vi "CharToByte(SubVI).vi"(9 "use char":bool, 10 "input u8":u8, 11 "input char":string) -> (1 "output asc":u8, 2 "output char":string, 3 "output u8":u8)   [LabVIEW 2012]
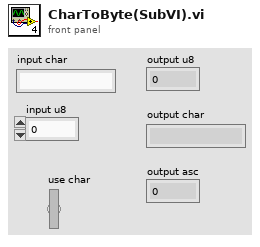
[diagram p1: front panel]
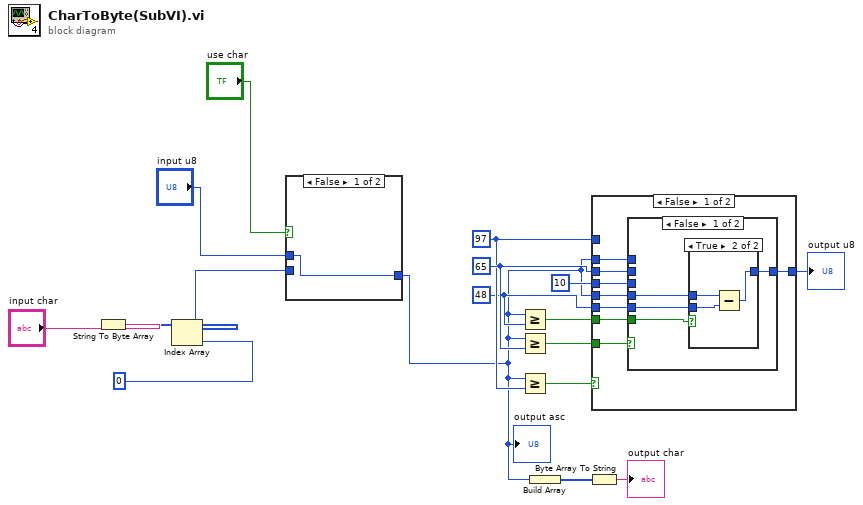
[diagram p0: block diagram]
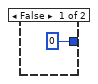
[diagram p3: hidden frame]
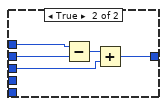
[diagram p4: hidden frame]
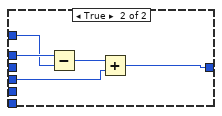
[diagram p5: hidden frame]
diagram:
  w13 = 48
  w17 = 65
  w16 = 97
  n1 = String To Byte Array(string="input char") -> (unsigned byte array=w7:u8[])
  n2 = Index Array(array=w7, index=0) -> (element=w3:u8)
  n3 = case shown="False" "use char" {
    tunnel: w3 -> [_ w19]
    tunnel: [w18 w19] -> w2
    tunnel: "input u8" -> [w18 _]
    frame False {
    }
    frame True {
    }
  }
  "output asc" <- w2
  n4 = Greater Or Equal?(x=w2, y=w13) -> (x >= y?=w12:bool)
  n5 = Greater Or Equal?(x=w2, y=w17) -> (x >= y?=w14:bool)
  n6 = Greater Or Equal?(x=w2, y=w16) -> (x >= y?=w15:bool)
  n7 = Build Array(w2) -> (w11:u8[])
  n8 = Byte Array To String(unsigned byte array=w11) -> (string=→"output char":string)
  n9 = case shown="False" w15 {
    tunnel: w14 -> [w27 _]
    tunnel: w12 -> [w26 _]
    tunnel: w2 -> [w20 w45]
    tunnel: w16 -> [_ w44]
    tunnel: 10 -> [w22 w43]
    tunnel: [w25 w41] -> w6
    tunnel: w2 -> [w24 _]
    tunnel: w13 -> [w23 _]
    tunnel: w17 -> [w21 _]
    frame False {
      n10 = case shown="False" w27 {
        tunnel: w26 -> [w31 _]
        tunnel: [w30 w40] -> w25
        tunnel: w24 -> [w29 _]
        tunnel: w23 -> [w28 _]
        tunnel: w22 -> [_ w39]
        tunnel: w21 -> [_ w37]
        tunnel: w20 -> [_ w36]
        frame False {
          n11 = case shown="True" w31 {
            tunnel: [0 w33] -> w30
            tunnel: w29 -> [_ w35]
            tunnel: w28 -> [_ w34]
            frame False {
            }
            frame True {
              n12 = Subtract(x=w35, y=w34) -> (x-y=w33:i32)
            }
          }
        }
        frame True {
          n13 = Subtract(x=w36, y=w37) -> (x-y=w38:i32)
          n14 = Add(x=w38, y=w39) -> (x+y=w40:i32)
        }
      }
    }
    frame True {
      n15 = Subtract(x=w45, y=w44) -> (x-y=w42:i32)
      n16 = Add(x=w42, y=w43) -> (x+y=w41:i32)
    }
  }
  "output u8" <- w6
